vi "Read Device Identification.vi"(8 "error in (no error)":errorcluster, 9 "object ID":u8, 10 "read device ID code":T2=1 items=["Basic"=1, "Regular"=2, "Extended"=3, "Single"=4], 11 "MB session in":refnum<class "MB_Master.lvclass">) -> (0 "error out":errorcluster, 1 "Conformity Level":u8, 2 "DevID Objects":T1[](array[typedef]), 3 "MB session out":refnum<class "MB_Master.lvclass">)   [LabVIEW 2021, in "MB Master.lvlib"]
doc: "Function Code 43 / 14: Read device ID objects. Specify the type of access using the <b>read device ID code</b> and the id of the starting object using <b>object ID</b>.\n\nread device ID codes:\n 0x01 - Basic: Request the basic stream of devID objects (0x00 to 0x02) starting from the specified object ID.\n 0x02 - Regular: Requests the regular stream of devID objects (0x00 to 0x7F) starting from the specified object ID.\n 0x03 - Extended: Requests the extended stream of devID objects (0x00 to 0xFF) starting from the specified object ID.\n 0x04 - Single: Requests a single devID object specified by object ID.\n\nResponse is an array of devID objects. Each element contains the object ID and string value. The conformity level indicates the type of access supported by the device.\n\nConformity level values:\n0x01 - Basic (stream only)\n0x02 - Regular (stream only)\n0x03 - Extended (stream only)\n0x81 - Basic (stream and single)\n0x82 - Regular (stream and single)\n0x83 - Extended (stream and single)"
uses:
  <vilib>/Plasmionique/MB Master/MB Master.lvlib
  <vilib>/Plasmionique/MB Master/MB_Master/MB_Master.lvclass
  <vilib>/Plasmionique/MB Master/MB_PDU/MB_ReadDevID Codes.ctl
  <vilib>/Plasmionique/MB Master/MB_PDU/MB_DevID Object.ctl
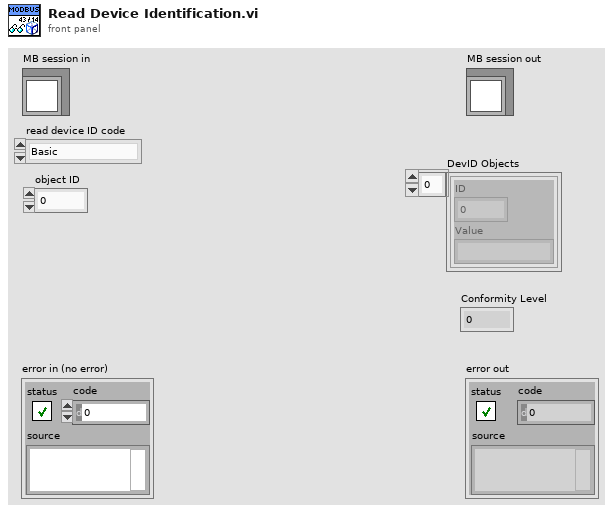
[diagram p1: front panel]
types:
  T1 = typedef "MB Master.lvlib/MB_DevID Object.ctl" = cluster{"ID":u8, "Value":string}
  T2 = typedef "MB Master.lvlib/MB_ReadDevID Codes.ctl" = u8
  T3 = typedef "MB Master.lvlib/MB_PDU_Cluster.ctl" = cluster{"Function Code":u8, "Data":u8[], "RTU_DataBytes":i32}
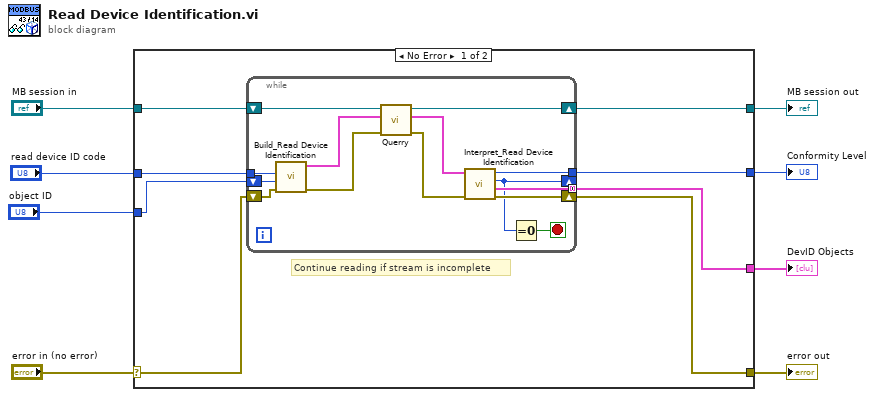
[diagram p0: block diagram]
diagram:
  n1 = case shown="No Error" "error in (no error)" {
    selector: "error in (no error)" -> [w14 w32]
    tunnel: [w11 w32] -> w7
    tunnel: [w16 w31] -> w5
    tunnel: "MB session in" -> [w15 w31]
    tunnel: "read device ID code" -> [w13 _]
    tunnel: "object ID" -> [w12 _]
    tunnel: [w10 _] -> w2
    tunnel: [w9 _] -> w1
    frame No Error {
      # "Continue reading if stream is incomplete"
      n2 = while {
        tunnel: w13 -> [w26]
        tunnel: [w20] -> w10 mode=concatenating
        tunnel: [w19] -> w9
        shift-right: [w18] -> _
        shift-left: w12 -> [w25]
        shift-right: [w21] -> w11
        shift-left: w14 -> [w27]
        shift-right: [w30] -> w16
        shift-left: w15 -> [w29]
        stop <- w17 stop-if-true
        n3 = call <vilib>:"Build_Read Device Identification.vi"("error in (no error)"=w27, "object ID"=w25, "read device ID code"=w26) -> ("error out"=w28:errorcluster, "MB_PDU"=w24:T3)  [unwired: 7 in]
        n4 = call-dynamic "Querry.vi"("error in (no error)"=w28, "PDU_req"=w24, "MB_Master in"=w29) -> ("error out"=w22:errorcluster, "PDU_resp"=w23:T3, "MB_Master out"=w30:refnum<class "MB_Master.lvclass">)  [unwired: 6 in]
        n5 = call <vilib>:"Interpret_Read Device Identification.vi"("error in (no error)"=w22, "MB_PDU_resp in"=w23) -> ("error out"=w21:errorcluster, "DevID Objects"=w20:T1[], "Next Object ID"=w18:u8, "Conformity Level"=w19:u8)  [unwired: 6 in]
        n6 = Equal To 0?(x=w18) -> (x = 0?=w17:bool)
      }
    }
    frame Error {
    }
  }
  "error out" <- w7
  "MB session out" <- w5
  "DevID Objects" <- w2
  "Conformity Level" <- w1
